vi "Observe Data.vi"(6 "Time Stamp":timestamp, 8 "error in (no error)":errorcluster, 9 "Value":variant, 10 "Datum Name":string, 11 "Normal Active Station View in":refnum<class "Normal Active Option View.lvclass">) -> (0 "error out":errorcluster, 3 "Normal Active Station View out":refnum<class "Normal Active Option View.lvclass">)   [LabVIEW 2019, in "Normal Active Option View.lvclass"]
doc: "<License>\nCopyright © 2017 Composed Systems, LLC | All rights reserved\nwww.composed.io\n\nAuthor: Ethan Stern <ethan.stern@composed.io>\n\nThis software is provided \"AS IS\" WITHOUT WARRANTIES, either express or implied, AND IS FOR EDUCATIONAL PURPOSES ONLY.\n</License>"
uses:
  <vilib>/gpm_packages/@cs/Car-wash/Source/Normal Active Station View/Normal Active Station View/Normal Active Option View.lvclass
  <vilib>/gpm_packages/@cs/Car-wash/Source/Normal Active Station View/Normal Active Station View/Normal Active Option View.lvclass/Normal Active Option View.ctl
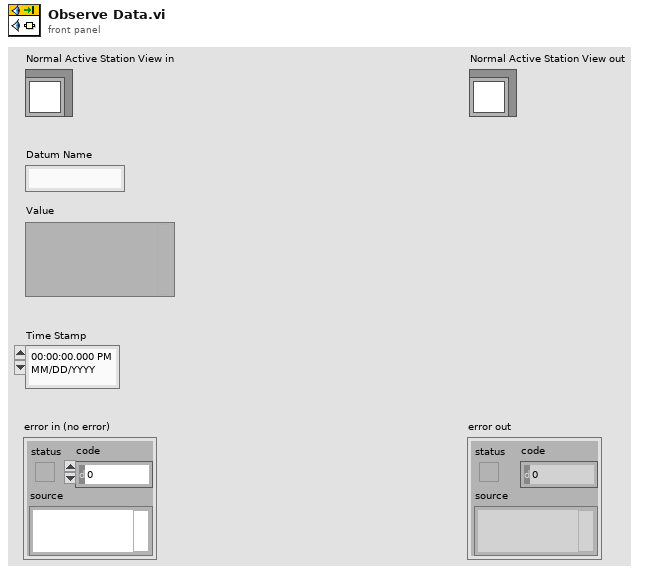
[diagram p1: front panel]
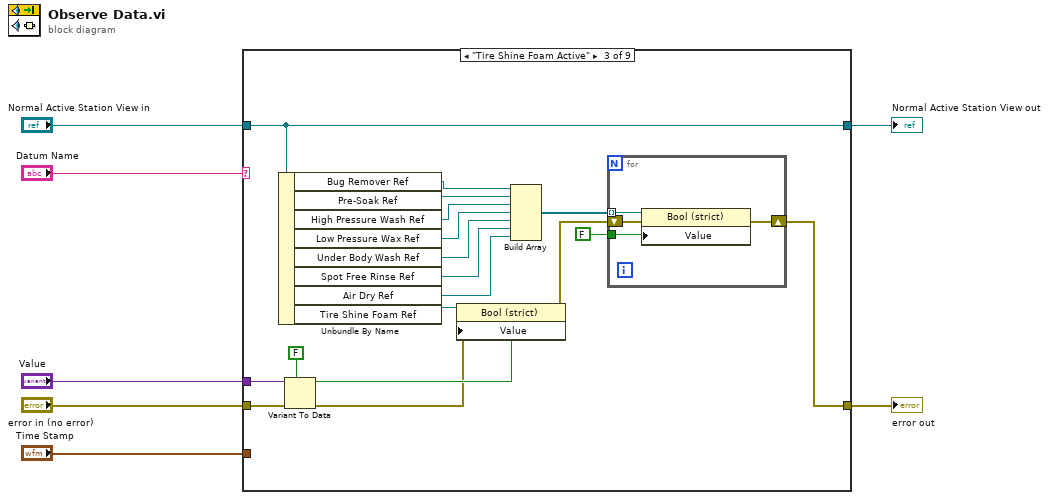
[diagram p0: block diagram]
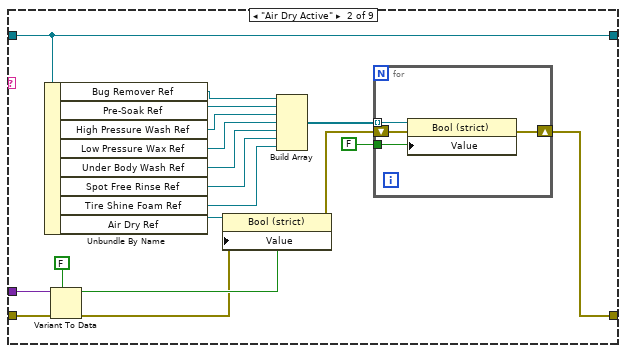
[diagram p3: hidden frame]
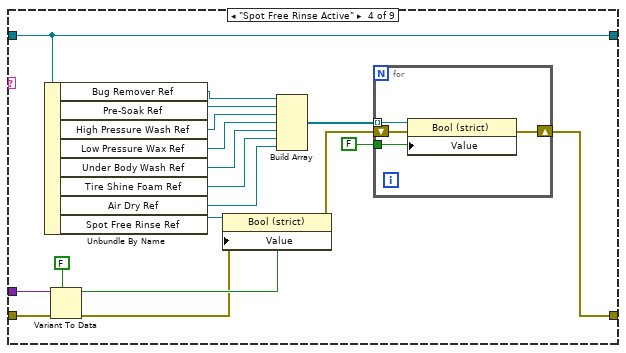
[diagram p4: hidden frame]
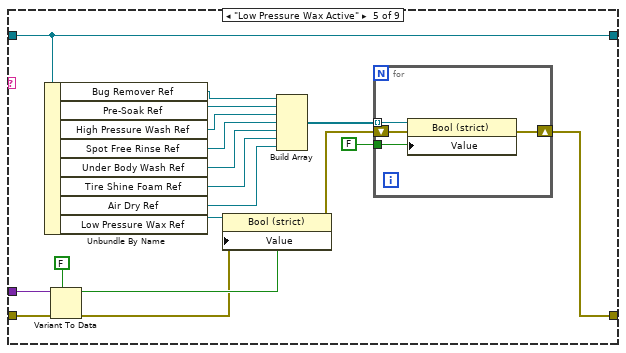
[diagram p5: hidden frame]
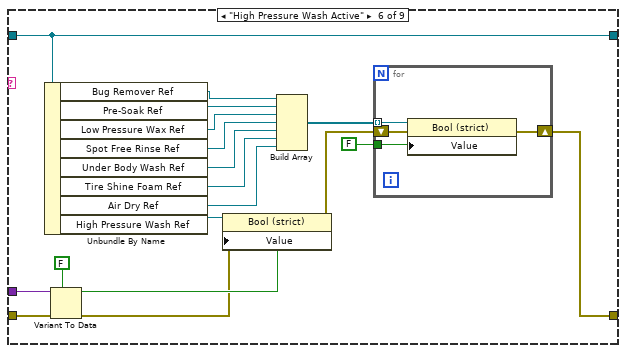
[diagram p6: hidden frame]
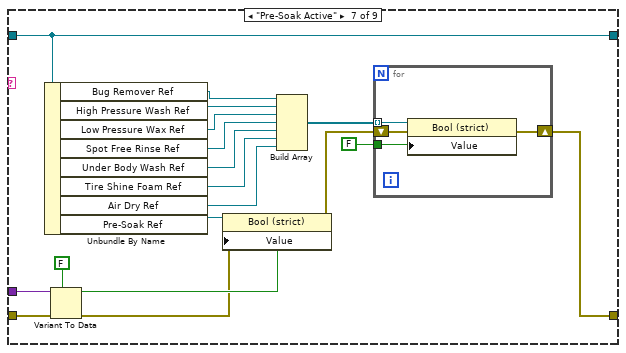
[diagram p7: hidden frame]
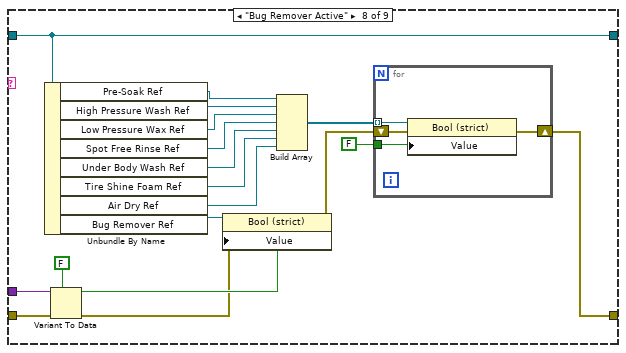
[diagram p8: hidden frame]
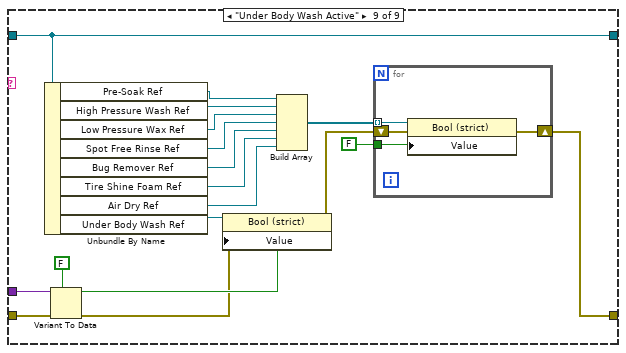
[diagram p9: hidden frame]
diagram:
  n1 = case shown="\"Tire Shine Foam Active\"" "Datum Name" {
    tunnel: "Normal Active Station View in" -> [w8 w27 w49 w71 w93 w115 w137 w159 w181]
    tunnel: "Value" -> [_ w19 w41 w63 w85 w107 w129 w151 w173]
    tunnel: "error in (no error)" -> [w9 w18 w40 w62 w84 w106 w128 w150 w172]
    tunnel: "Time Stamp" -> [_ _ _ _ _ _ _ _ _]
    tunnel: [w8 w27 w49 w71 w93 w115 w137 w159 w181] -> w2
    tunnel: [w9 w10 w32 w54 w76 w98 w120 w142 w164] -> w1
    frame Default {
    }
    frame "Air Dry Active" {
      n2 = Unbundle By Name(w27) -> ("Bug Remover Ref"=w26:refnum<vi>, "Pre-Soak Ref"=w25:refnum<vi>, "High Pressure Wash Ref"=w24:refnum<vi>, "Low Pressure Wax Ref"=w23:refnum<vi>, "Under Body Wash Ref"=w22:refnum<vi>, "Spot Free Rinse Ref"=w21:refnum<vi>, "Tire Shine Foam Ref"=w20:refnum<vi>, "Air Dry Ref"=w16:refnum<vi>)
      n3 = Variant To Data(error in=w18, type=FALSE, Variant=w19) -> (data=w15:bool, error out=w12:errorcluster)
      n4 = property class="Bool (strict)"(reference=w16, error in=w12, "Value"=w15) -> (error out=w11:errorcluster)  [unwired: 1 out]
      n5 = Build Array(w26, w25, w24, w23, w22, w21, w20) -> (w14:refnum<vi>[])
      n6 = for {
        tunnel: w14 -> [w31] mode=indexing
        tunnel: FALSE -> [w30]
        shift-right: [w28] -> w10
        shift-left: w11 -> [w29]
        n7 = property class="Bool (strict)"(reference=w31, error in=w29, "Value"=w30) -> (error out=w28:errorcluster)  [unwired: 1 out]
      }
    }
    frame "Tire Shine Foam Active" {
      n8 = Unbundle By Name(w49) -> ("Bug Remover Ref"=w48:refnum<vi>, "Pre-Soak Ref"=w47:refnum<vi>, "High Pressure Wash Ref"=w46:refnum<vi>, "Low Pressure Wax Ref"=w45:refnum<vi>, "Under Body Wash Ref"=w44:refnum<vi>, "Spot Free Rinse Ref"=w43:refnum<vi>, "Air Dry Ref"=w42:refnum<vi>, "Tire Shine Foam Ref"=w38:refnum<vi>)
      n9 = Variant To Data(error in=w40, type=FALSE, Variant=w41) -> (data=w37:bool, error out=w34:errorcluster)
      n10 = property class="Bool (strict)"(reference=w38, error in=w34, "Value"=w37) -> (error out=w33:errorcluster)  [unwired: 1 out]
      n11 = Build Array(w48, w47, w46, w45, w44, w43, w42) -> (w36:refnum<vi>[])
      n12 = for {
        tunnel: w36 -> [w53] mode=indexing
        tunnel: FALSE -> [w52]
        shift-right: [w50] -> w32
        shift-left: w33 -> [w51]
        n13 = property class="Bool (strict)"(reference=w53, error in=w51, "Value"=w52) -> (error out=w50:errorcluster)  [unwired: 1 out]
      }
    }
    frame "Spot Free Rinse Active" {
      n14 = Unbundle By Name(w71) -> ("Bug Remover Ref"=w70:refnum<vi>, "Pre-Soak Ref"=w69:refnum<vi>, "High Pressure Wash Ref"=w68:refnum<vi>, "Low Pressure Wax Ref"=w67:refnum<vi>, "Under Body Wash Ref"=w66:refnum<vi>, "Tire Shine Foam Ref"=w65:refnum<vi>, "Air Dry Ref"=w64:refnum<vi>, "Spot Free Rinse Ref"=w60:refnum<vi>)
      n15 = Variant To Data(error in=w62, type=FALSE, Variant=w63) -> (data=w59:bool, error out=w56:errorcluster)
      n16 = property class="Bool (strict)"(reference=w60, error in=w56, "Value"=w59) -> (error out=w55:errorcluster)  [unwired: 1 out]
      n17 = Build Array(w70, w69, w68, w67, w66, w65, w64) -> (w58:refnum<vi>[])
      n18 = for {
        tunnel: w58 -> [w75] mode=indexing
        tunnel: FALSE -> [w74]
        shift-right: [w72] -> w54
        shift-left: w55 -> [w73]
        n19 = property class="Bool (strict)"(reference=w75, error in=w73, "Value"=w74) -> (error out=w72:errorcluster)  [unwired: 1 out]
      }
    }
    frame "Low Pressure Wax Active" {
      n20 = Unbundle By Name(w93) -> ("Bug Remover Ref"=w92:refnum<vi>, "Pre-Soak Ref"=w91:refnum<vi>, "High Pressure Wash Ref"=w90:refnum<vi>, "Spot Free Rinse Ref"=w89:refnum<vi>, "Under Body Wash Ref"=w88:refnum<vi>, "Tire Shine Foam Ref"=w87:refnum<vi>, "Air Dry Ref"=w86:refnum<vi>, "Low Pressure Wax Ref"=w82:refnum<vi>)
      n21 = Variant To Data(error in=w84, type=FALSE, Variant=w85) -> (data=w81:bool, error out=w78:errorcluster)
      n22 = property class="Bool (strict)"(reference=w82, error in=w78, "Value"=w81) -> (error out=w77:errorcluster)  [unwired: 1 out]
      n23 = Build Array(w92, w91, w90, w89, w88, w87, w86) -> (w80:refnum<vi>[])
      n24 = for {
        tunnel: w80 -> [w97] mode=indexing
        tunnel: FALSE -> [w96]
        shift-right: [w94] -> w76
        shift-left: w77 -> [w95]
        n25 = property class="Bool (strict)"(reference=w97, error in=w95, "Value"=w96) -> (error out=w94:errorcluster)  [unwired: 1 out]
      }
    }
    frame "High Pressure Wash Active" {
      n26 = Unbundle By Name(w115) -> ("Bug Remover Ref"=w114:refnum<vi>, "Pre-Soak Ref"=w113:refnum<vi>, "Low Pressure Wax Ref"=w112:refnum<vi>, "Spot Free Rinse Ref"=w111:refnum<vi>, "Under Body Wash Ref"=w110:refnum<vi>, "Tire Shine Foam Ref"=w109:refnum<vi>, "Air Dry Ref"=w108:refnum<vi>, "High Pressure Wash Ref"=w104:refnum<vi>)
      n27 = Variant To Data(error in=w106, type=FALSE, Variant=w107) -> (data=w103:bool, error out=w100:errorcluster)
      n28 = property class="Bool (strict)"(reference=w104, error in=w100, "Value"=w103) -> (error out=w99:errorcluster)  [unwired: 1 out]
      n29 = Build Array(w114, w113, w112, w111, w110, w109, w108) -> (w102:refnum<vi>[])
      n30 = for {
        tunnel: w102 -> [w119] mode=indexing
        tunnel: FALSE -> [w118]
        shift-right: [w116] -> w98
        shift-left: w99 -> [w117]
        n31 = property class="Bool (strict)"(reference=w119, error in=w117, "Value"=w118) -> (error out=w116:errorcluster)  [unwired: 1 out]
      }
    }
    frame "Pre-Soak Active" {
      n32 = Unbundle By Name(w137) -> ("Bug Remover Ref"=w136:refnum<vi>, "High Pressure Wash Ref"=w135:refnum<vi>, "Low Pressure Wax Ref"=w134:refnum<vi>, "Spot Free Rinse Ref"=w133:refnum<vi>, "Under Body Wash Ref"=w132:refnum<vi>, "Tire Shine Foam Ref"=w131:refnum<vi>, "Air Dry Ref"=w130:refnum<vi>, "Pre-Soak Ref"=w126:refnum<vi>)
      n33 = Variant To Data(error in=w128, type=FALSE, Variant=w129) -> (data=w125:bool, error out=w122:errorcluster)
      n34 = property class="Bool (strict)"(reference=w126, error in=w122, "Value"=w125) -> (error out=w121:errorcluster)  [unwired: 1 out]
      n35 = Build Array(w136, w135, w134, w133, w132, w131, w130) -> (w124:refnum<vi>[])
      n36 = for {
        tunnel: w124 -> [w141] mode=indexing
        tunnel: FALSE -> [w140]
        shift-right: [w138] -> w120
        shift-left: w121 -> [w139]
        n37 = property class="Bool (strict)"(reference=w141, error in=w139, "Value"=w140) -> (error out=w138:errorcluster)  [unwired: 1 out]
      }
    }
    frame "Bug Remover Active" {
      n38 = Unbundle By Name(w159) -> ("Pre-Soak Ref"=w158:refnum<vi>, "High Pressure Wash Ref"=w157:refnum<vi>, "Low Pressure Wax Ref"=w156:refnum<vi>, "Spot Free Rinse Ref"=w155:refnum<vi>, "Under Body Wash Ref"=w154:refnum<vi>, "Tire Shine Foam Ref"=w153:refnum<vi>, "Air Dry Ref"=w152:refnum<vi>, "Bug Remover Ref"=w148:refnum<vi>)
      n39 = Variant To Data(error in=w150, type=FALSE, Variant=w151) -> (data=w147:bool, error out=w144:errorcluster)
      n40 = property class="Bool (strict)"(reference=w148, error in=w144, "Value"=w147) -> (error out=w143:errorcluster)  [unwired: 1 out]
      n41 = Build Array(w158, w157, w156, w155, w154, w153, w152) -> (w146:refnum<vi>[])
      n42 = for {
        tunnel: w146 -> [w163] mode=indexing
        tunnel: FALSE -> [w162]
        shift-right: [w160] -> w142
        shift-left: w143 -> [w161]
        n43 = property class="Bool (strict)"(reference=w163, error in=w161, "Value"=w162) -> (error out=w160:errorcluster)  [unwired: 1 out]
      }
    }
    frame "Under Body Wash Active" {
      n44 = Unbundle By Name(w181) -> ("Pre-Soak Ref"=w180:refnum<vi>, "High Pressure Wash Ref"=w179:refnum<vi>, "Low Pressure Wax Ref"=w178:refnum<vi>, "Spot Free Rinse Ref"=w177:refnum<vi>, "Bug Remover Ref"=w176:refnum<vi>, "Tire Shine Foam Ref"=w175:refnum<vi>, "Air Dry Ref"=w174:refnum<vi>, "Under Body Wash Ref"=w170:refnum<vi>)
      n45 = Variant To Data(error in=w172, type=FALSE, Variant=w173) -> (data=w169:bool, error out=w166:errorcluster)
      n46 = property class="Bool (strict)"(reference=w170, error in=w166, "Value"=w169) -> (error out=w165:errorcluster)  [unwired: 1 out]
      n47 = Build Array(w180, w179, w178, w177, w176, w175, w174) -> (w168:refnum<vi>[])
      n48 = for {
        tunnel: w168 -> [w185] mode=indexing
        tunnel: FALSE -> [w184]
        shift-right: [w182] -> w164
        shift-left: w165 -> [w183]
        n49 = property class="Bool (strict)"(reference=w185, error in=w183, "Value"=w184) -> (error out=w182:errorcluster)  [unwired: 1 out]
      }
    }
  }
  "error out" <- w1
  "Normal Active Station View out" <- w2
